vi "EnabledChannelArray.vi"(8 "Channel3":i16, 9 "Channel2":i16, 10 "Channel1":i16, 11 "Channel0":i16) -> (3 "EnabledChannels":string[](array[string]))   [LabVIEW 2020]
uses:
  shared/OnOffTypeDef.ctl
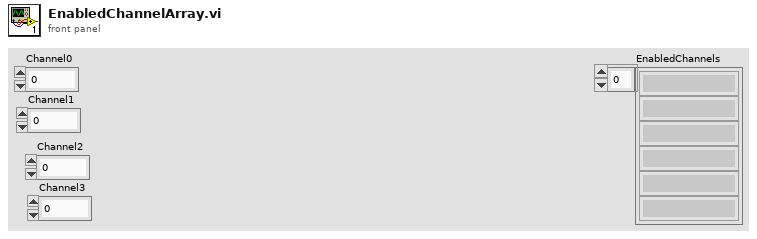
[diagram p1: front panel]
types:
  T1 = typedef "OnOffTypeDef.ctl" = enum16{"off", "on"}
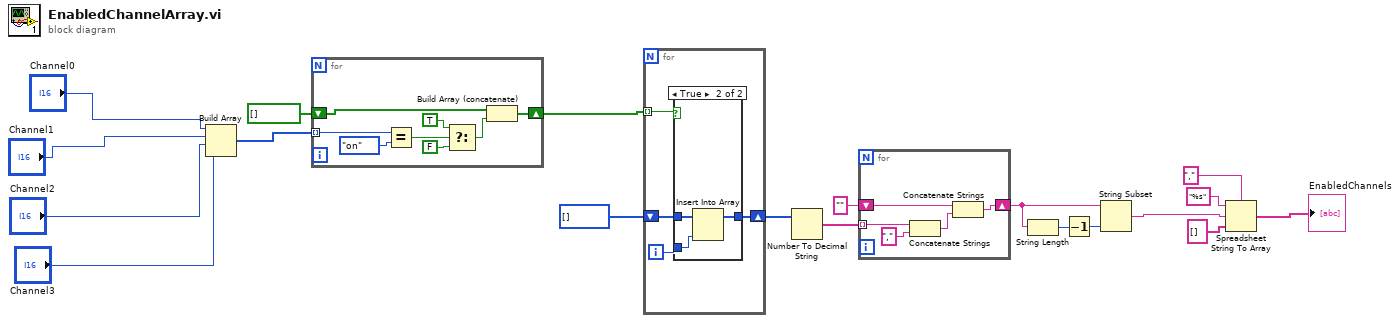
[diagram p0: block diagram]
diagram:
  n1 = Build Array("Channel0", "Channel1", "Channel2", "Channel3") -> (w9:i16[])
  n2 = for {
    tunnel: w9 -> [w27] mode=indexing
    shift-right: [w20] -> w8
    shift-left: bool[] [] -> [w22]
    n3 = Equal?(x=w27, y=OnOffTypeDef."on" ("Settings.channelenabled.Channel0")) -> (x = y?=w25:bool)
    n4 = Select(t=TRUE, s=w25, f=FALSE) -> (s? t:f=w21:bool)
    n5 = Build Array (concatenate)(w22, w21) -> (w20:bool[])
  }
  n6 = for {
    tunnel: w8 -> [w31] mode=indexing
    shift-right: [w29] -> w6
    shift-left: i32[] [] -> [w30]
    i -> [w28]
    n7 = case shown="True" w31 {
      tunnel: [w32 w35] -> w29
      tunnel: w30 -> [w32 w34]
      tunnel: w28 -> [_ w33]
      frame False {
      }
      frame True {
        n8 = Insert Into Array(array=w34, new element=w33) -> (w35:i32[])  [unwired: 1 in]
      }
    }
  }
  n9 = Number To Decimal String(number=w6) -> (decimal integer string=w18:string[])  [unwired: 1 in]
  n10 = for {
    tunnel: w18 -> [w39] mode=indexing
    shift-right: [w38] -> w17
    shift-left: "" -> [w37]
    n11 = Concatenate Strings(w39, "," ("string")) -> (w36:string)
    n12 = Concatenate Strings(w37, w36) -> (w38:string)
  }
  n13 = String Length(string=w17) -> (length=w15:i32)
  n14 = Decrement(x=w15) -> (x-1=w16:i32)
  n15 = String Subset(string=w17, length (rest)=w16) -> (substring=w19:string)  [unwired: 1 in]
  n16 = Spreadsheet String To Array(delimiter (Tab)=",", format string="%s", spreadsheet string=w19, array type (2D Dbl)=string[] []) -> (array=→"EnabledChannels":string[])
